vi "SerialFINAL.vi"() -> ()   [LabVIEW 2020]
uses:
  <vilib>/Instr/_visa.llb/VISA Configure Serial Port (Instr).vi
  <vilib>/ErrorRing/Error Ring.xnode
panel:
  out "Waveform Chart 2":cluster{dbl, dbl}(graph)
  out "Waveform Chart":cluster{dbl, dbl}(graph)
  out "VOTAJES":dbl[](array[slide]) scale=0.0..5.0
  in  "LED 4":bool
  in  "LED 3":bool
  in  "LED 2":bool
  in  "LED 1":bool
  in  "stop":bool
  out "IN DIGI":i32[](array[numeric])
  out "ADC":i32[](array[numeric])
  out "read buffer":string
  in  "PUERTO":refnum<visa-resource-name>
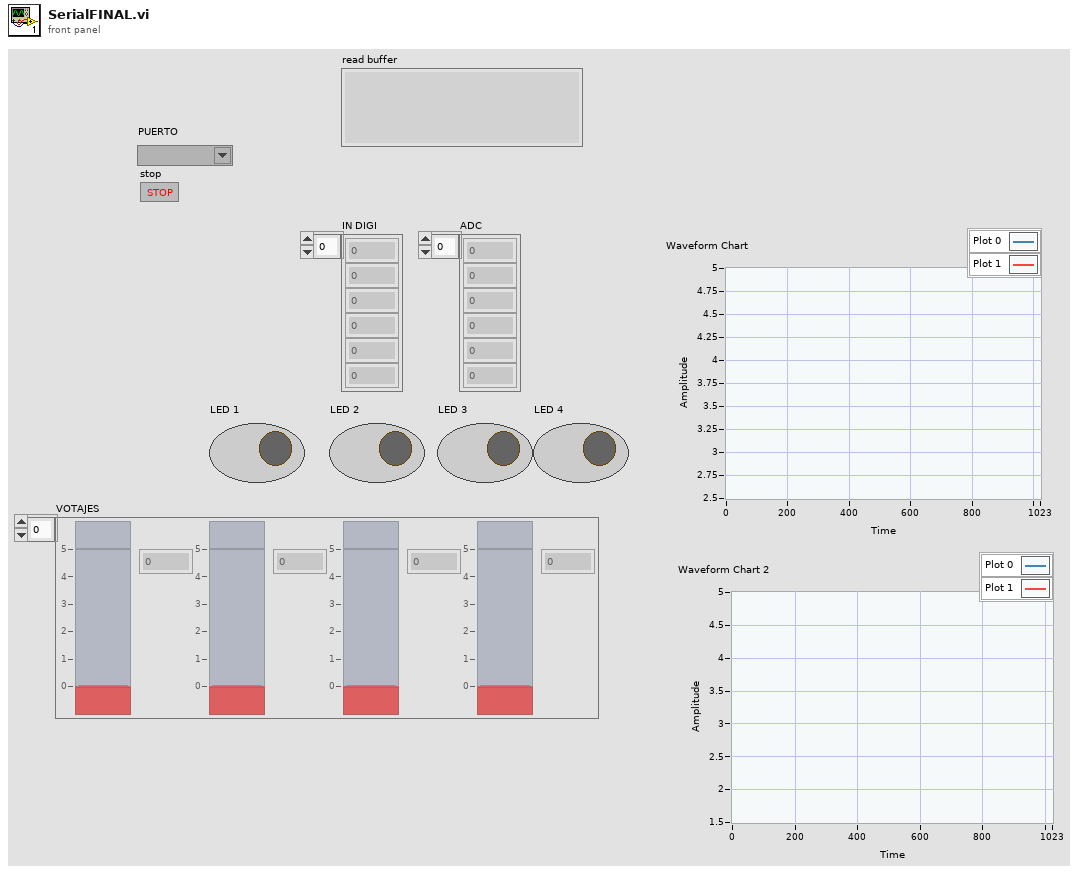
[diagram p1: front panel]
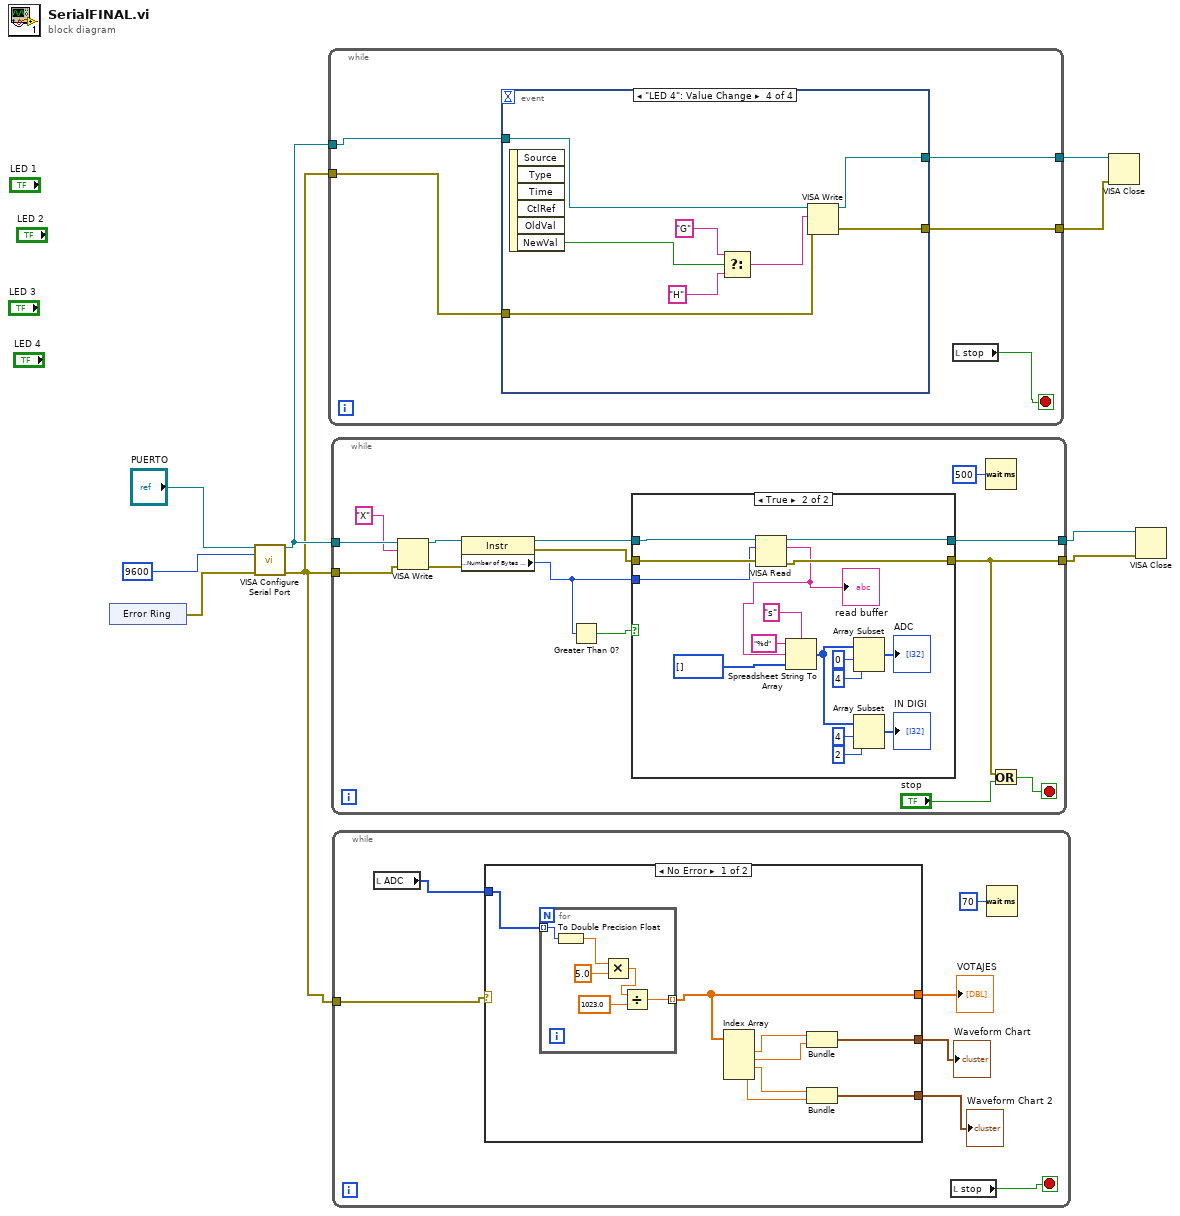
[diagram p0: block diagram]
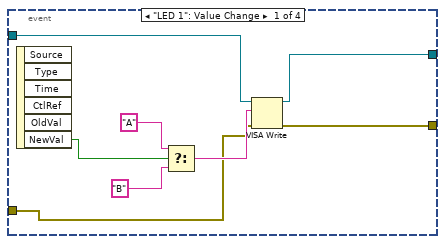
[diagram p2: hidden frame]
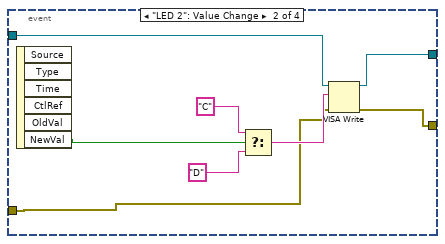
[diagram p3: hidden frame]
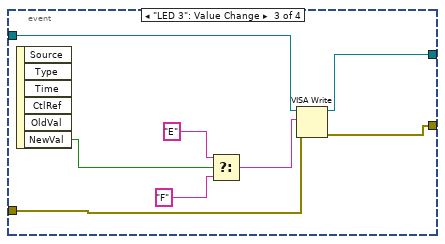
[diagram p4: hidden frame]
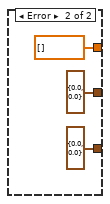
[diagram p5: hidden frame]
diagram:
  n1 = xnode "Error Ring"() -> ("error out"=w7:errorcluster)
  n2 = call-poly "VISA Configure Serial Port"("VISA resource name"="PUERTO", "baud rate (9600)"=u32 9600, "error in (no error)"=w7) -> ("VISA resource name out"=w4:refnum<visa-resource-name>, "error out"=w1:errorcluster)  [unwired: 11 in]
  n3 = while {
    tunnel: w4 -> [w14]
    tunnel: w1 -> [w13]
    tunnel: [w12] -> w3
    tunnel: [w11] -> w2
    stop <- w10 stop-if-true
    n4 = event shown="[3] \"LED 4\": Value Change" {
      selector: _ -> [_ _ _ _]
      dyn-events: _ -> [_ _ _ _]
      timeout: _ -> [_ _ _ _]
      tunnel: w14 -> [w18 w25 w35 w43]
      tunnel: w13 -> [w17 w26 w34 w42]
      tunnel: [w16 w24 w33 w41] -> w12
      tunnel: [w15 w23 w32 w40] -> w11
      event "LED 1": Value Change {
        n5 = event-data() -> ("NewVal"=w20:bool)  [unwired: 1 in, 5 out]
        n6 = Select(t="A", s=w20, f="B") -> (s? t:f=w19:string)
        n7 = VISA Write(VISA resource name=w18, write buffer=w19, error in (no error)=w17) -> (VISA resource name out=w16:refnum<visa-resource-name>, error out=w15:errorcluster)  [unwired: 1 out]
      }
      event "LED 2": Value Change {
        n8 = event-data() -> ("NewVal"=w27:bool)  [unwired: 1 in, 5 out]
        n9 = Select(t="C", s=w27, f="D") -> (s? t:f=w30:string)
        n10 = VISA Write(VISA resource name=w25, write buffer=w30, error in (no error)=w26) -> (VISA resource name out=w24:refnum<visa-resource-name>, error out=w23:errorcluster)  [unwired: 1 out]
      }
      event "LED 3": Value Change {
        n11 = event-data() -> ("NewVal"=w31:bool)  [unwired: 1 in, 5 out]
        n12 = Select(t="E", s=w31, f="F") -> (s? t:f=w38:string)
        n13 = VISA Write(VISA resource name=w35, write buffer=w38, error in (no error)=w34) -> (VISA resource name out=w33:refnum<visa-resource-name>, error out=w32:errorcluster)  [unwired: 1 out]
      }
      event "LED 4": Value Change {
        n14 = event-data() -> ("NewVal"=w39:bool)  [unwired: 1 in, 5 out]
        n15 = Select(t="G", s=w39, f="H") -> (s? t:f=w46:string)
        n16 = VISA Write(VISA resource name=w43, write buffer=w46, error in (no error)=w42) -> (VISA resource name out=w41:refnum<visa-resource-name>, error out=w40:errorcluster)  [unwired: 1 out]
      }
    }
    n17 = local read "stop"() -> (w10:bool)
  }
  n18 = while {
    tunnel: w4 -> [w60]
    tunnel: w1 -> [w59]
    tunnel: [w51] -> w6
    tunnel: [w49] -> w5
    stop <- w50 stop-if-true
    n19 = VISA Write(VISA resource name=w60, write buffer="X", error in (no error)=w59) -> (VISA resource name out=w57:refnum<visa-resource-name>, error out=w56:errorcluster)  [unwired: 1 out]
    n20 = property class="Instr"(reference=w57, error in=w56) -> (reference out=w54:refnum<visa-resource-name>, error out=w53:errorcluster, "Serial Settings:Number of Bytes at Serial Port"=w52:u32)
    n21 = Greater Than 0?(x=w52) -> (x > 0?=w55:bool)
    n22 = case shown="True" w55 {
      tunnel: [w62 w75] -> w51
      tunnel: w54 -> [w62 w78]
      tunnel: [w61 w74] -> w49
      tunnel: w53 -> [w61 w77]
      tunnel: w52 -> [_ w76]
      frame False {
      }
      frame True {
        n23 = VISA Read(VISA resource name=w78, byte count=w76, error in (no error)=w77) -> (VISA resource name out=w75:refnum<visa-resource-name>, read buffer=w73:string, error out=w74:errorcluster)  [unwired: 1 out]
        "read buffer" <- w73
        n24 = Spreadsheet String To Array(delimiter (Tab)="s", format string="%d", spreadsheet string=w73, array type (2D Dbl)=i32[] []) -> (array=w69:i32[])
        n25 = Array Subset(array=w69, index=0, length=4) -> (→"ADC":i32[])
        n26 = Array Subset(array=w69, index=4, length=2) -> (→"IN DIGI":i32[])
      }
    }
    n27 = Wait (ms)(milliseconds to wait=u32 500) -> ()  [unwired: 1 out]
    n28 = Or(x=w49, y="stop") -> (x .or. y?=w50:bool)
  }
  n29 = while {
    tunnel: w1 -> [w84]
    stop <- w85 stop-if-true
    n30 = local read "ADC"() -> (w83:i32[])
    n31 = case shown="No Error" w84 {
      tunnel: w83 -> [w93 _]
      tunnel: [w92 dbl[] []] -> w82
      tunnel: [w87 cluster{dbl, dbl} {0.0, 0.0}] -> w81
      tunnel: [w86 cluster{dbl, dbl} {0.0, 0.0}] -> w80
      frame No Error {
        n32 = for {
          tunnel: w93 -> [w99] mode=indexing
          tunnel: [w94] -> w92 mode=indexing
          n33 = To Double Precision Float(number=w99) -> (double precision float=w98:dbl)
          n34 = Multiply(x=w98, y=5.0) -> (x*y=w96:dbl)
          n35 = Divide(x=w96, y=1023.0) -> (x/y=w94:dbl)
        }
        n36 = Index Array(array=w92) -> (element #1=w91:dbl, element #2=w90:dbl, element #3=w89:dbl, element #4=w88:dbl)  [unwired: 4 in]
        n37 = Bundle(w91, w90) -> (w87:cluster{dbl, dbl})  [unwired: 1 in]
        n38 = Bundle(w89, w88) -> (w86:cluster{dbl, dbl})  [unwired: 1 in]
      }
      frame Error {
      }
    }
    "VOTAJES" <- w82
    "Waveform Chart" <- w81
    "Waveform Chart 2" <- w80
    n39 = local read "stop"() -> (w85:bool)
    n40 = Wait (ms)(milliseconds to wait=u32 70) -> ()  [unwired: 1 out]
  }
  n41 = VISA Close(VISA resource name=w3, error in (no error)=w2) -> ()  [unwired: 1 out]
  n42 = VISA Close(VISA resource name=w6, error in (no error)=w5) -> ()  [unwired: 1 out]
